vi "Test Get-Set Data Name.vi"(8 "error in (no error)":errorcluster) -> (0 "error out":errorcluster, 3 "Passed":bool)   [LabVIEW 2020]
uses:
  <vilib>/addons/_JKI Toolkits/Caraya/classes/Assert/Assert.lvclass
  <vilib>/addons/_JKI Toolkits/Caraya/classes/Test/Test.lvclass
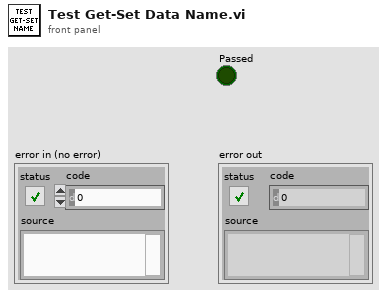
[diagram p1: front panel]
types:
  T1 = typedef "Type Descriptor Header.ctl" = cluster{"length":u16, "private":u8, "type":T2, "# elements":u16}
  T2 = typedef "Type Descriptor Enumeration.ctl" = enum8{"<Null>", "I8", "I16", "I32", "I64", "U8", "U16", "U32", "U64", "SGL", "DBL", "EXT", "CSG", "CDB", "CXT", "0x0F", "0x10", "0x11", "0x12", "0x13", "0x14", "Enum U8", "Enum U16", "Enum U32", "Enum U64", "SGL PQ", "DBL PQ", "EXT PQ", "CSG PQ", "CDB PQ", "CXT PQ", "0x1F", "0x20", "Boolean", "0x22", "0x23", "0x24", "0x25", "0x26", "0x27", "0x28", "0x29", "0x2A", "0x2B", "0x2C", "0x2D", "0x2E", "0x2F", "String", "0x31", "Path", "Pict", "0x34", "0x35", "0x36", "DAQ", "0x38", "0x39", "0x3A", "0x3B", "0x3C", "0x3D", "0x3E", "0x3F", "Array", "0x41", "0x42", "0x43", "0x44", "0x45", "0x46", "0x47", "0x48", "0x49", "0x4A", "0x4B", "0x4C", "0x4D", "0x4E", "0x4F", "Cluster", "0x51", "0x52", "Variant", "Waveform", "0x55", "0x56", "0x57", "0x58", "0x59", "0x5A", "0x5B", "0x5C", "0x5D", "0x5E", "Fixed Point", "0x60", "0x61", "0x62", "0x63", "0x64", "0x65", "0x66", "0x67", "0x68", "0x69", "0x6A", "0x6B", "0x6C", "0x6D", "0x6E", "0x6F", "Refnum", "0x71", "0x72", "Set Collection", "Map Collection"}
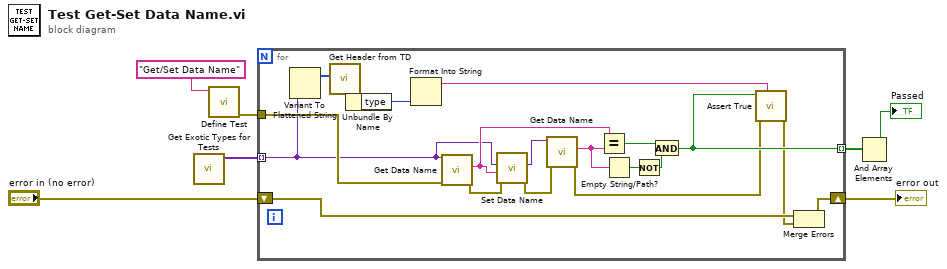
[diagram p0: block diagram]
diagram:
  n1 = call "Get Exotic Types for Tests.vi"() -> ("exotic types"=w1:variant[])  [unwired: 11 in]
  n2 = call <vilib>:"Define Test.vi"("Label (VI Title)"="Get/Set Data Name") -> ("error out"=w7:errorcluster)  [unwired: 10 in]
  n3 = for {
    tunnel: w1 -> [w12] mode=indexing
    shift-right: [w14] -> w2
    shift-left: "error in (no error)" -> [w16]
    tunnel: [w18] -> w4 mode=indexing
    tunnel: w7 -> [w13]
    n4 = Variant To Flattened String(Variant=w12) -> (1:w11:i16[])  [unwired: 1 out]
    n5 = call "Get Header from TD.vi"("Type Descriptor"=w11) -> ("Type Descriptor Header"=w10:T1)
    n6 = Unbundle By Name(w10) -> ("type"=w9:T2)
    n7 = Format Into String(w9) -> (resulting string=w8:string)  [unwired: 3 in, 1 out]
    n8 = call "Get Data Name.vi"("error in (no error)"=w13, "Data"=w12) -> ("error out"=w26:errorcluster, "Data Name"=w23:string)  [unwired: 7 in, 1 out]
    n9 = call "Set Data Name.vi"("error in (no error)"=w26, "Data Name"=w23, "Data"=w12) -> ("error out"=w25:errorcluster, "Renamed Data"=w24:variant)  [unwired: 7 in]
    n10 = call "Get Data Name.vi"("error in (no error)"=w25, "Data"=w24) -> ("error out"=w17:errorcluster, "Data Name"=w21:string)  [unwired: 7 in, 1 out]
    n11 = Equal?(x=w23, y=w21) -> (x = y?=w22:bool)
    n12 = Empty String/Path?(string/path=w21) -> (empty?=w20:bool)
    n13 = Not(x=w20) -> (.not. x?=w19:bool)
    n14 = And(x=w22, y=w19) -> (x .and. y?=w18:bool)
    n15 = call <vilib>:"Assert True.vi"("Label"=w8, "error in (no error)"=w17, "True?"=w18) -> ("error out"=w15:errorcluster)  [unwired: 8 in]
    n16 = Merge Errors(w16, w15) -> (w14:errorcluster)
  }
  "error out" <- w2
  n17 = And Array Elements(Boolean array=w4) -> (logical AND=→"Passed":bool)
